vi "saturate.vi"(9 "Upper Limit (10)":fxp<+/-,25,5>[](array[numeric])=[10.0, 10.0, 10.0, 10.0, 10.0], 10 "Lower Limit (-10)":fxp<+/-,25,5>[](array[numeric])=[-10.0, -10.0, -10.0, -10.0, -10.0], 11 "Array In":fxp<+/-,25,5>[](array[numeric])=[0.0, 0.0, 0.0, 0.0, 0.0]) -> (3 "Array Out":fxp<+/-,25,5>[](array[numeric]))   [LabVIEW 2020, in "Controller.lvlib"]
doc: "Saturation block\noutput = min(max(input,lower limit), min(upper limit, max(input,lower limit)))"
uses:
  Controller.lvlib
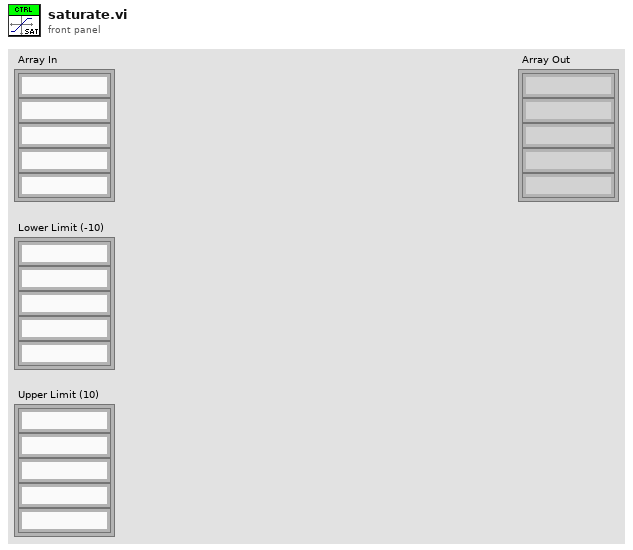
[diagram p1: front panel]
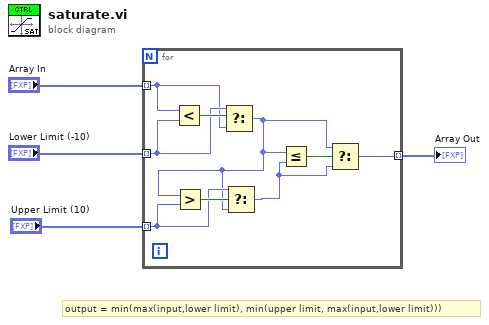
[diagram p0: block diagram]
diagram:
  # "output = min(max(input,lower limit), min(upper limit, max(input,lower limit)))"
  n1 = for {
    tunnel: "Array In" -> [w9] mode=indexing
    tunnel: "Lower Limit (-10)" -> [w10] mode=indexing
    tunnel: "Upper Limit (10)" -> [w12] mode=indexing
    tunnel: [w6] -> w1 mode=indexing
    n2 = Less?(x=w9, y=w10) -> (x < y?=w11:bool)
    n3 = Select(t=w10, s=w11, f=w9) -> (s? t:f=w5:fxp<+/-,25,5>)
    n4 = Greater?(x=w5, y=w12) -> (0:w13:bool)
    n5 = Select(t=w12, s=w13, f=w5) -> (s? t:f=w7:fxp<+/-,25,5>)
    n6 = Less Or Equal?(x=w5, y=w7) -> (x <= y?=w8:bool)
    n7 = Select(t=w5, s=w8, f=w7) -> (s? t:f=w6:fxp<+/-,25,5>)
  }
  "Array Out" <- w1
